vi "Initialize.vi"(8 "error in":errorcluster, 9 "Path":path, 10 "Device":string, 11 "Instruments in":refnum<class "Instruments.lvclass">) -> (0 "error out":errorcluster, 3 "Instruments out":refnum<class "Instruments.lvclass">)   [LabVIEW 2023, in "Instruments.lvlib" / "Instruments.lvclass"]
uses:
  Library/Instruments.lvclass
  Custom Controls/ConfigurationKeys.ctl
  Library/Instruments.lvclass/Instruments.ctl
  builds/Tools/Config.lvlibp/Config.lvclass
  C:/Users/Public/Documents/Development/builds/Tools/Config.lvlibp/Config.lvclass
  C:/Users/Public/Documents/Development/builds/Engine/Engine.lvlibp/Project/Engine.lvclass
  builds/Engine/Engine.lvlibp/Project/Engine.lvclass
panel:
  in  "Configuration Keys":T1
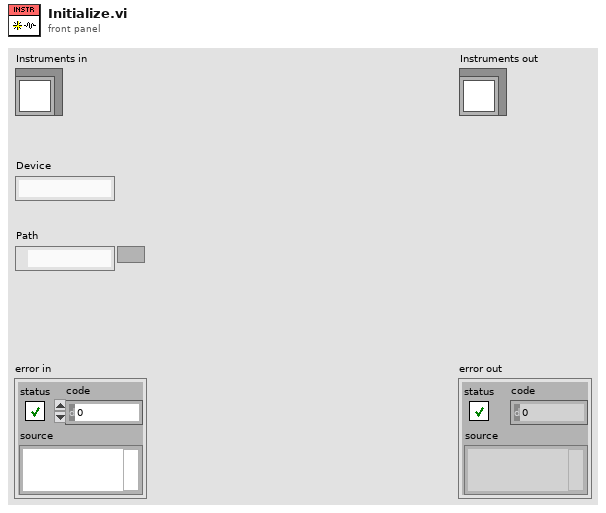
[diagram p1: front panel]
types:
  T1 = typedef "Instruments.lvlib/Instruments.lvclass/ConfigurationKeys.ctl" = enum16{"Calibration", "Resource", "Poll(ms)", "Panel", "Simulated", "Enabled"}
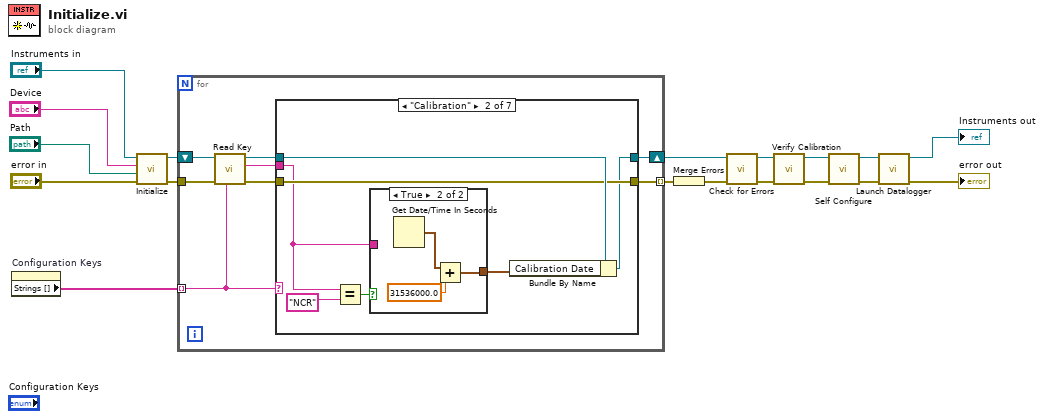
[diagram p0: block diagram]
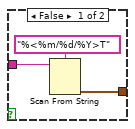
[diagram p3: hidden frame]
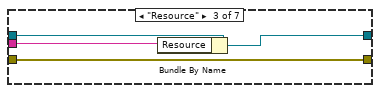
[diagram p4: hidden frame]
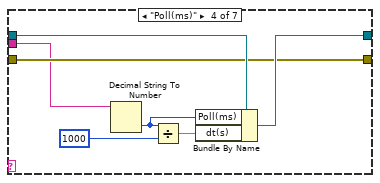
[diagram p5: hidden frame]
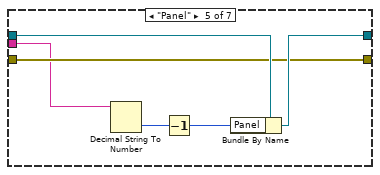
[diagram p6: hidden frame]
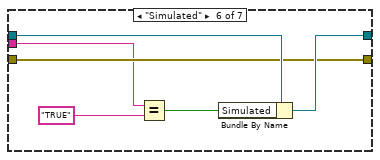
[diagram p7: hidden frame]
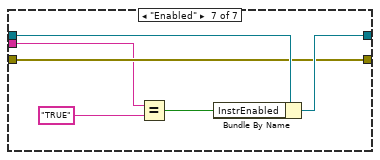
[diagram p8: hidden frame]
diagram:
  n1 = property on="Configuration Keys" class="Enum (strict)"() -> ("Strings []"=w9:string[])  [unwired: 2 in, 2 out]
  n2 = call-parent "Initialize.vi"("error in"="error in", "Path"="Path", "Device"="Device", "Config in"="Instruments in") -> ("error out"=w12:errorcluster, "Config out"=w13:refnum<class "Instruments.lvclass">)  [unwired: 6 in]
  n3 = for {
    tunnel: w9 -> [w21] mode=indexing
    shift-right: [w23] -> w6
    shift-left: w13 -> [w26]
    tunnel: w12 -> [w25]
    tunnel: [w19] -> w11 mode=indexing
    n4 = call "Read Key.vi"("Key Name"=w21, "error in"=w25, "Config in"=w26) -> ("error out"=w22:errorcluster, "Key Value"=w20:string, "Config out"=w24:refnum<class "Instruments.lvclass">)  [unwired: 6 in]
    n5 = case shown="\"Calibration\"" w21 {
      tunnel: w24 -> [w28 w35 w45 w52 w58 w64 w70]
      tunnel: [w28 w33 w44 w51 w57 w63 w69] -> w23
      tunnel: w22 -> [w27 w34 w42 w50 w56 w62 w68]
      tunnel: w20 -> [_ w30 w43 w49 w55 w61 w67]
      tunnel: [w27 w34 w42 w50 w56 w62 w68] -> w19
      frame "False", Default {
      }
      frame "Calibration" {
        n6 = Equal?(x=w30, y="NCR") -> (x = y?=w29:bool)
        n7 = case shown="True" w29 {
          tunnel: [w37 w41] -> w32
          tunnel: w30 -> [w36 _]
          frame False {
            n8 = Scan From String(format string="%<%m/%d/%Y>T", input string=w36) -> (output 1=w37:timestamp)  [unwired: 3 in, 3 out]
          }
          frame True {
            n9 = Get Date/Time In Seconds() -> (seconds since 1Jan1904=w40:timestamp)
            n10 = Add(x=w40, y=31536000.0) -> (x+y=w41:timestamp)
          }
        }
        n11 = Bundle By Name(cluster=w35, "Calibration Date"=w32) -> (w33:refnum<class "Instruments.lvclass">)
      }
      frame "Resource" {
        n12 = Bundle By Name(cluster=w45, "Resource"=w43) -> (w44:refnum<class "Instruments.lvclass">)
      }
      frame "Poll(ms)" {
        n13 = Decimal String To Number(string=w49) -> (number=w46:i32)  [unwired: 2 in, 1 out]
        n14 = Divide(x=w46, y=1000) -> (x/y=w47:dbl)
        n15 = Bundle By Name(cluster=w52, "Poll(ms)"=w46, "dt(s)"=w47) -> (w51:refnum<class "Instruments.lvclass">)
      }
      frame "Panel" {
        n16 = Decimal String To Number(string=w55) -> (number=w54:i32)  [unwired: 2 in, 1 out]
        n17 = Decrement(x=w54) -> (x-1=w53:i32)
        n18 = Bundle By Name(cluster=w58, "Panel"=w53) -> (w57:refnum<class "Instruments.lvclass">)
      }
      frame "Simulated" {
        n19 = Equal?(x=w61, y="TRUE") -> (x = y?=w60:bool)
        n20 = Bundle By Name(cluster=w64, "Simulated"=w60) -> (w63:refnum<class "Instruments.lvclass">)
      }
      frame "Enabled" {
        n21 = Equal?(x=w67, y="TRUE") -> (x = y?=w66:bool)
        n22 = Bundle By Name(cluster=w70, "InstrEnabled"=w66) -> (w69:refnum<class "Instruments.lvclass">)
      }
    }
  }
  n23 = Merge Errors(w11) -> (w5:errorcluster)
  n24 = call "Check for Errors.vi"("error in"=w5, "Engine in"=w6) -> ("error out"=w4:errorcluster, "Engine out"=w3:refnum<class "Instruments.lvclass">)  [unwired: 8 in]
  n25 = call "Verify Calibration.vi"("error in"=w4, "Instruments in"=w3) -> ("error out"=w8:errorcluster, "Instruments out"=w7:refnum<class "Instruments.lvclass">)  [unwired: 8 in]
  n26 = call-dynamic "Self Configure.vi"("error in"=w8, "Instruments in"=w7) -> ("error out"=w17:errorcluster, "Instruments out"=w18:refnum<class "Instruments.lvclass">)  [unwired: 8 in]
  n27 = call "Launch Datalogger.vi"("error in"=w17, "Instruments in"=w18) -> ("error out"=→"error out":errorcluster, "Instruments out"=→"Instruments out":refnum<class "Instruments.lvclass">)  [unwired: 8 in]
